vi "Create CNG Provider.vi"(8 "error in (no error)":errorcluster, 11 "Crypto Provider":T1) -> (0 "error out":errorcluster, 3 "CngProvider":refnum<k24>)   [LabVIEW 2021, in "dotNET Crypto Key Management.lvlib"]
doc: "Create an instance of a .NET Crypto Provider from either the MS Software Key Provider or Platform Provider (Hardware based - TPM)."
uses:
  dotNET Crypto Key Management.lvlib
  System.Core
  CNG Provider Type.ctl
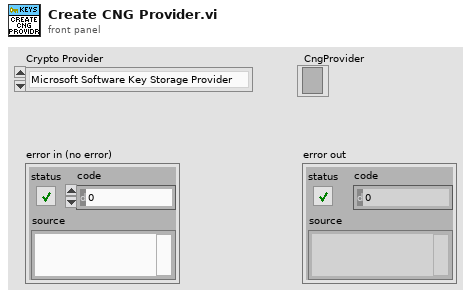
[diagram p1: front panel]
types:
  T1 = typedef "dotNET Crypto Key Management.lvlib/CNG Provider Type.ctl" = enum16{"Microsoft Software Key Storage Provider", "Microsoft Platform Crypto Provider"}
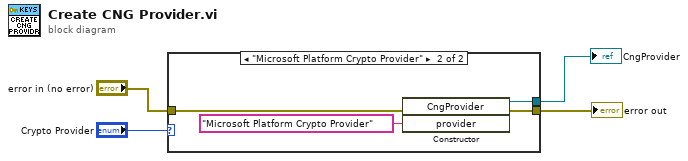
[diagram p0: block diagram]
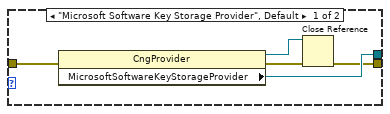
[diagram p2: hidden frame]
diagram:
  n1 = case shown="\"Microsoft Platform Crypto Provider\"" "Crypto Provider" {
    tunnel: [w9 w12] -> w2
    tunnel: "error in (no error)" -> [w7 w11]
    tunnel: [w6 w10] -> w4
    frame "Microsoft Software Key Storage Provider", Default {
      n2 = property class="CngProvider"(error in=w7) -> (reference out=w5:refnum<k24>, error out=w8:errorcluster, "MicrosoftSoftwareKeyStorageProvider"=w9:refnum<k24>)  [unwired: 1 in]
      n3 = Close Reference(reference=w5, error in (no error)=w8) -> (error out=w6:errorcluster)
    }
    frame "Microsoft Platform Crypto Provider" {
      n4 = constructor class="CngProvider"(error in=w11, "provider"="Microsoft Platform Crypto Provider") -> (reference out=w12:refnum<k24>, error out=w10:errorcluster)  [unwired: 2 in, 2 out]
    }
  }
  "error out" <- w4
  "CngProvider" <- w2
